vi "2 NoSailGoodness.vi"(9 "Waypoint in":refnum<class "Waypoint.lvclass">, 10 "Heading to Test":dbl) -> (2 "Goodness":dbl)   [LabVIEW 2011]
doc: "Gives a goodness value to a test heading based on how it avoids no sail zones. All no sail zones of the current waypoint are considered. \n\nOutputs a value between 0 and 1 where 1 means the boat is not facing any no sail zones (they are more than 90 degrees away from the test heading) and 0 means the boat will go directly into a no sail zone if it maintains that test heading."
uses:
  2 Globals/2 Global.vi
  2 Classes/Waypoint/Waypoint.lvclass
  2 Globals/2 TuningConstants.vi
  2 Typedefs/UTM Circle.ctl
  2 Typedefs/UTM Location.ctl
panel:
  out "Robot UTM Location":T1 {"North" format="%#_10f"; "East" format="%#_8f"}
  out "No-sail circles considered":T2[](array[typedef])
  out "Tuning Quotient":dbl=0.05 step=0.1
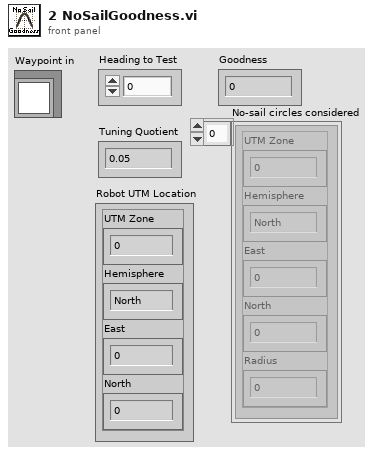
[diagram p1: front panel]
types:
  T1 = typedef "UTM Location.ctl" = cluster{"UTM Zone":dbl, "Hemisphere":enum16{"North", "South"}, "East":dbl, "North":dbl}
  T2 = typedef "UTM Circle.ctl" = cluster{"UTM Zone":dbl, "Hemisphere":enum16{"North", "South"}, "East":dbl, "North":dbl, "Radius":dbl}
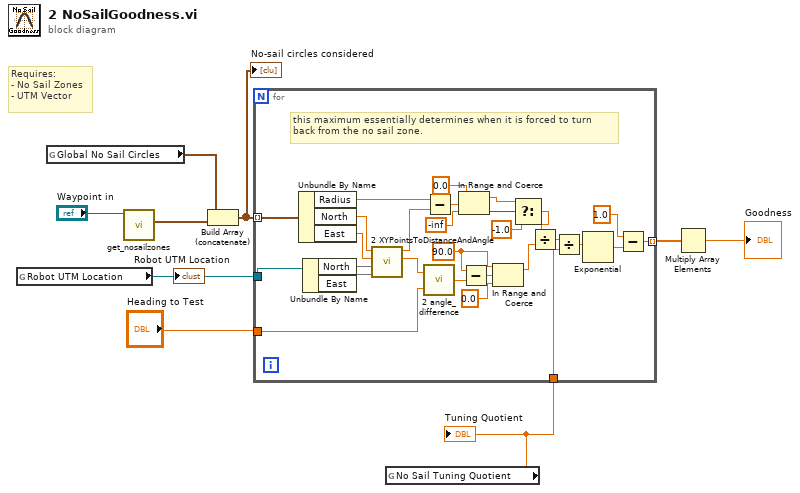
[diagram p0: block diagram]
diagram:
  # "Requires:\n- No Sail Zones\n- UTM Vector"
  n1 = global read "2 Global.vi" "Robot UTM Location"() -> (w8:refnum<class "UTM_Location.lvclass">)
  "Robot UTM Location" <- w8
  n2 = global read "2 Global.vi" "Global No Sail Circles"() -> (w5:T2[])
  n3 = call-dynamic "get_nosailzones.vi"("Waypoint in"="Waypoint in") -> ("No Sail Circles"=w4:T2[])  [unwired: 7 in, 2 out]
  n4 = Build Array (concatenate)(w5, w4) -> (w3:T2[])
  "No-sail circles considered" <- w3
  n5 = global read "2 TuningConstants.vi" "No Sail Tuning Quotient"() -> (w2:dbl)
  "Tuning Quotient" <- w2
  n6 = for {
    tunnel: "Heading to Test" -> [w31]
    tunnel: w3 -> [w37] mode=indexing
    tunnel: w8 -> [w36]
    tunnel: [w25] -> w7 mode=indexing
    tunnel: w2 -> [w16]
    w19 = 90.0
    # "this maximum essentially determines when it is forced to turn\nback from the no sail zone."
    n7 = Unbundle By Name(w37) -> ("Radius"=w30:dbl, "North"=w35:dbl, "East"=w34:dbl)
    n8 = Unbundle By Name(w36) -> ("North"=w33, "East"=w32)
    n9 = call "2 XYPointsToDistanceAndAngle.vi"("East 2"=w32, "North 2"=w33, "East 1"=w34, "North 1"=w35) -> ("Angle Diff"=w11:dbl, "Distance"=w29:dbl)  [unwired: 6 in]
    n10 = call "2 angle_difference.vi"("Angle 2"=w31, "Angle 1"=w11) -> ("Difference"=w24:dbl)
    n11 = Subtract(x=w30, y=w29) -> (x-y=w28:dbl)
    n12 = In Range and Coerce(upper limit=0.0, x=w28, lower limit=-inf) -> (coerced(x)=w14:dbl, In Range?=w15:bool)
    n13 = Subtract(x=w19, y=w24) -> (x-y=w23:dbl)
    n14 = In Range and Coerce(upper limit=w19, x=w23, lower limit=0.0) -> (coerced(x)=w21:dbl)  [unwired: 1 out]
    n15 = Select(t=w14, s=w15, f=-1.0) -> (s? t:f=w13:dbl)
    n16 = Divide(x=w13, y=w21) -> (x/y=w18:dbl)
    n17 = Divide(x=w18, y=w16) -> (x/y=w17:dbl)
    n18 = Exponential(1:w17) -> (0:w27:dbl)
    n19 = Subtract(x=1.0, y=w27) -> (x-y=w25:dbl)
  }
  n20 = Multiply Array Elements(1:w7) -> (0:→"Goodness":dbl)
